vi "CLD 8 CSV file commands utility Exercise.vi"(8 "Error In":errorcluster) -> (0 "Error Out":errorcluster, 3 "Commands Out Array":T1[](array[typedef]))   [LabVIEW 2025]
doc: "CLD 8 exercise"
uses:
  CLD 8 Data Cluster.ctl
  <vilib>/Utility/file.llb/Read Delimited Spreadsheet (string).vi
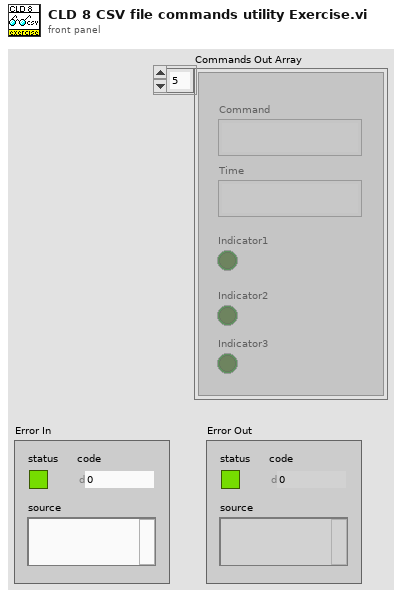
[diagram p1: front panel]
types:
  T1 = typedef "CLD 8 Data Cluster.ctl" = cluster{"Command":string, "Time":string, "Indicator1":bool, "Indicator2":bool, "Indicator3":bool}
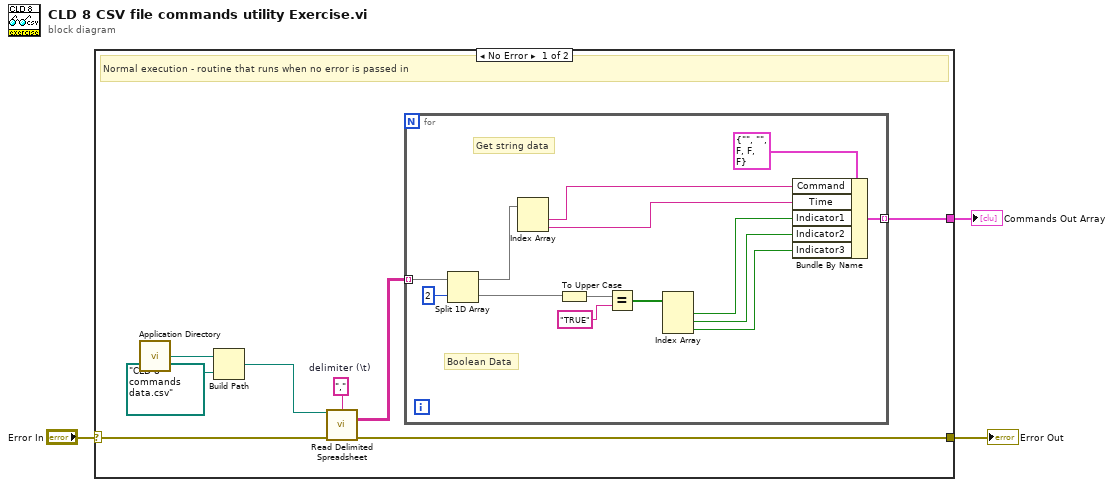
[diagram p0: block diagram]
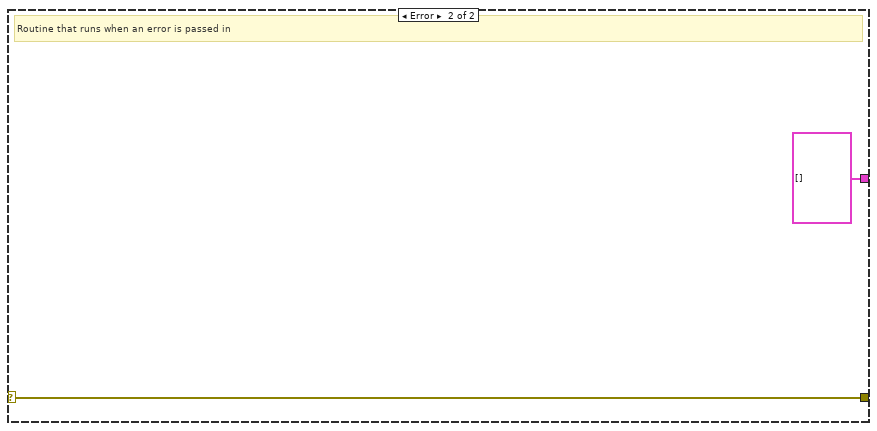
[diagram p2: hidden frame]
diagram:
  n1 = case shown="No Error" "Error In" {
    selector: "Error In" -> [w11 w27]
    tunnel: [w10 w27] -> w2
    tunnel: [w5 T1[] []] -> w1
    frame No Error {
      w4 = ","  # delimiter (\t)
      # "Normal execution - routine that runs when no error is passed in"
      n2 = call <vilib>:"Application Directory.vi"() -> ("Application Directory"=w9:path)
      n3 = Build Path(base path=w9, name or relative path=path "CLD 8 commands data.csv") -> (appended path=w7:path)
      n4 = call-poly <vilib>:"Read Delimited Spreadsheet.vi"("file path (dialog if empty)"=w7, "error in (no error)"=w11, "delimiter (\\t)"=w4) -> ("all rows"=w6:string[][], "error out"=w10:errorcluster)  [unwired: 7 in, 4 out]
      n5 = for {
        tunnel: w6 -> [w23] mode=indexing
        tunnel: [w12] -> w5 mode=indexing
        # "Boolean Data"
        # "Get string data"
        n6 = Split 1D Array(array=w23, index=2) -> (first subarray=w20:string[], second subarray=w21:string[])
        n7 = Index Array(array=w20) -> (element #1=w24:string, element #2=w19:string)  [unwired: 2 in]
        n8 = To Upper Case(1:w21) -> (0:w18:string[])
        n9 = Equal?(x=w18, y="TRUE") -> (x = y?=w16:bool[])
        n10 = Index Array(array=w16) -> (element #1=w15:bool, element #2=w14:bool, element #3=w13:bool)  [unwired: 3 in]
        n11 = Bundle By Name(cluster=T1 {"Command"="", "Time"="", "Indicator1"=FALSE, "Indicator2"=FALSE, "Indicator3"=FALSE} ("Cluster 3"), "Command"=w24, "Time"=w19, "Indicator1"=w15, "Indicator2"=w14, "Indicator3"=w13) -> (w12:T1)
      }
    }
    frame Error {
      # "Routine that runs when an error is passed in"
    }
  }
  "Error Out" <- w2
  "Commands Out Array" <- w1
